vi "DrawRectangleOnImageARGB.vi"(4 "Thickness (Default: 1)":i32=1, 6 "ARGB Colour":T2={"Alpha"=255, "RGB"=0}, 7 "OpenCV Line Type (Default LINE_8)":T3=enum."LINE_8", 8 "error in (no error)":errorcluster, 9 "Point B":T1, 10 "Point A":T1, 11 "ARGB Image":refnum<data-value>) -> (0 "error out":errorcluster, 3 "ARGB Image (Duplicate)":refnum<data-value>)   [LabVIEW 2020, in "g_ar_toolkit.image.lvlib"]
uses:
  g_ar_toolkit.image.lvlib
  Line Type.ctl
  g_ar_toolkit.common/Image Point (Integer).ctl
  ARGB Colour.ctl
  <vilib>/Utility/error.llb/Error Cluster From Error Code.vi
  7e6fb015-3761-4366-a0a7-e436eb229083.vi
  g_ar_toolkit.common/g_ar_toolkit_common.lvlib
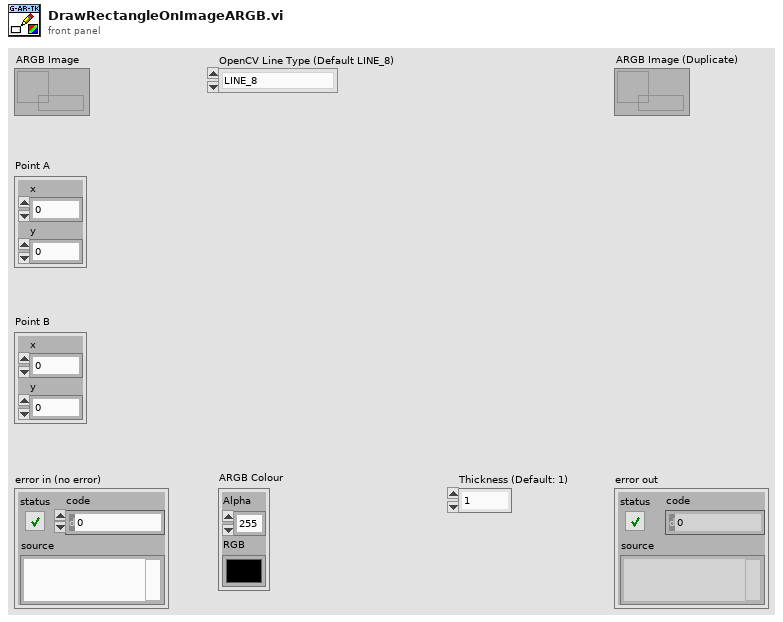
[diagram p1: front panel]
types:
  T1 = typedef "g_ar_toolkit_common.lvlib/Image Point (Integer).ctl" = cluster{"x":i32, "y":i32}
  T2 = typedef "g_ar_toolkit.image.lvlib/ARGB Colour.ctl" = cluster{"Alpha":u8, "RGB":u32}
  T3 = typedef "g_ar_toolkit.image.lvlib/Line Type.ctl" = enum8{"FILLED", "LINE_4", "LINE_8", "LINE_AA"}
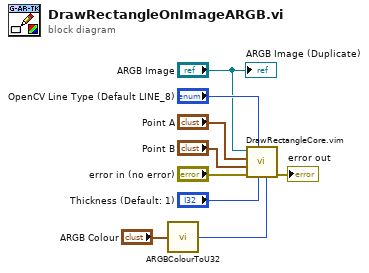
[diagram p0: block diagram]
diagram:
  n1 = call "ARGBColourToU32.vi"("ARGB Colour"="ARGB Colour") -> ("U32 Colour"=w3:u32)
  n2 = call "DrawRectangleCore.vim"("Colour"=w3, "Thickness"="Thickness (Default: 1)", "OpenCV Line Type"="OpenCV Line Type (Default LINE_8)", "error in (no error)"="error in (no error)", "Point B"="Point B", "Point A"="Point A", "Src"="ARGB Image") -> ("error out"=→"error out":errorcluster)  [unwired: 4 in]
  "ARGB Image (Duplicate)" <- "ARGB Image"
